vi "Query count display mode.vi"(8 "error in (no error)":errorcluster, 11 "VISA resource name":refnum<visa-resource-name>) -> (0 "error out":errorcluster, 2 "output":T1, 3 "VISA resource name out":refnum<visa-resource-name>)   [LabVIEW 2015, in "SR400.lvlib"]
doc: "SD { j }\nIf j = 1, the SD command sets the count display\nmode to HOLD. If j = 0, the display mode will be\nCONTINUOUS. If j is absent, the display mode is\nreturned."
uses:
  SR400.lvlib
  Typedefs/Display Mode.ctl
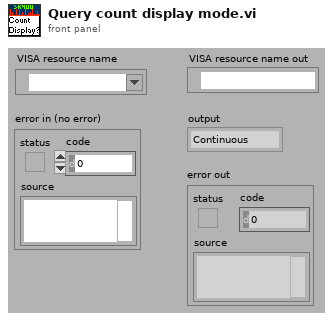
[diagram p1: front panel]
types:
  T1 = typedef "SR400.lvlib/Display Mode.ctl" = enum16{"Continuous", "Hold"}
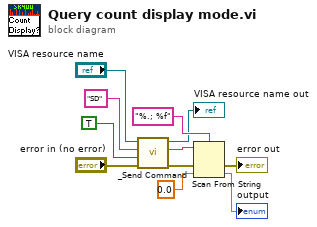
[diagram p0: block diagram]
diagram:
  n1 = call "_Send Command.vi"("error in (no error)"="error in (no error)", "Query? (F)"=TRUE, "Command"="SD" ("command"), "VISA resource name"="VISA resource name") -> ("error out"=w2:errorcluster, "Response"=w3:string, "VISA resource name out"=→"VISA resource name out":refnum<visa-resource-name>)  [unwired: 5 out]
  n2 = Scan From String(format string="%.; %f", input string=w3, error in=w2, default 1=0.0 ("default value 1")) -> (error out=→"error out":errorcluster, output 1=→"output":dbl)  [unwired: 1 in, 2 out]
